vi "CameraSubVI.vi"(2 "Plik wyjsciowy 2":path=path "f:/test.jpg") -> ()   [LabVIEW 2023]
uses:
  <vilib>/userDefined/High Color/IMAQdx.ctl
  <vilib>/vision/driver/NI_Vision_Acquisition_Software.lvlib
panel:
  out "Image 3":T1(plugin-control) caption="Image"
  in  "Zapisz 2":bool
  in  "stop 2":bool
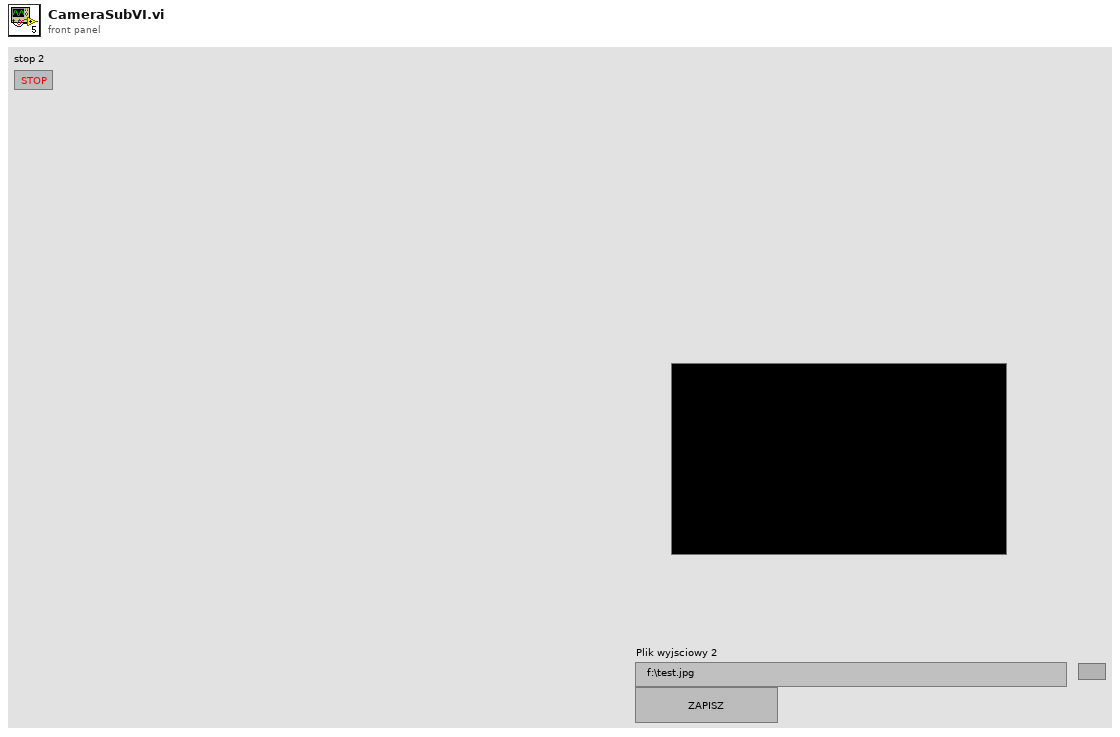
[diagram p1: front panel]
types:
  T1 = typedef "IMAQ Image.ctl" = refnum<image>
  T2 = typedef "IMAQdx.ctl" = refnum<k21>
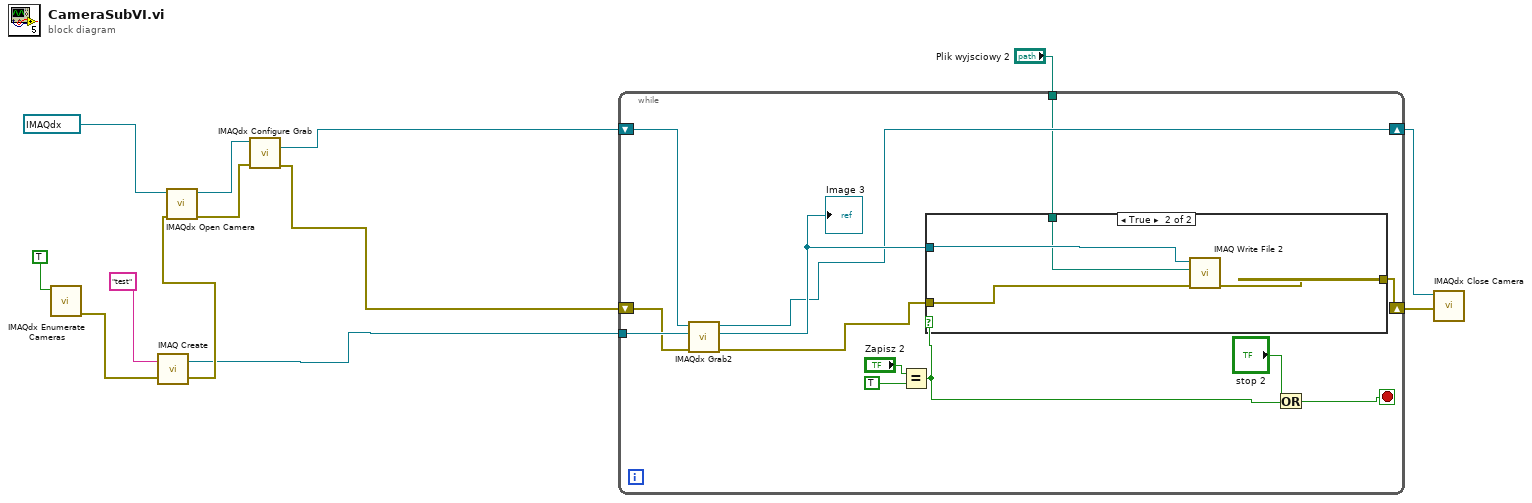
[diagram p0: block diagram]
diagram:
  n1 = call <vilib>:"IMAQdx Enumerate Cameras.vi"("Connected Only? (Yes)"=TRUE) -> ("error out"=w12:errorcluster)  [unwired: 9 in, 1 out]
  n2 = call "IMAQ Create"("Image Name"="test", "error in (no error)"=w12) -> ("New Image"=w8:T1, "error out"=w10:errorcluster)  [unwired: 2 in, 1 out]
  n3 = call <vilib>:"IMAQdx Open Camera.vi"("error in"=w10, "Session In"=T2 "cam0") -> ("error out"=w5:errorcluster, "Session Out"=w6:T2)  [unwired: 1 in, 7 out]
  n4 = call <vilib>:"IMAQdx Configure Grab.vi"("error in"=w5, "Session In"=w6) -> ("error out"=w4:errorcluster, "Session Out"=w3:T2)  [unwired: 8 in]
  n5 = while {
    tunnel: w8 -> [w22]
    shift-right: [w26] -> w9
    shift-left: w4 -> [w19]
    shift-right: [w20] -> w7
    shift-left: w3 -> [w18]
    tunnel: "Plik wyjsciowy 2" -> [w14]
    stop <- w15 stop-if-true
    n6 = call <vilib>:"IMAQdx Grab2.vi"("error in"=w19, "Image In"=w22, "Session In"=w18) -> ("error out"=w23:errorcluster, "Image Out"=w21:T1, "Session Out"=w20:T2)  [unwired: 5 in, 1 out]
    "Image 3" <- w21
    n7 = Equal?(x="Zapisz 2", y=TRUE) -> (x = y?=w17:bool)
    n8 = case shown="True" w17 {
      tunnel: w23 -> [w27 w31]
      tunnel: [w27 w30] -> w26
      tunnel: w21 -> [_ w29]
      tunnel: w14 -> [_ w28]
      frame False {
      }
      frame True {
        n9 = call-poly "IMAQ Write File 2"("error in (no error)"=w31, "File Path"=w28, "Image"=w29) -> ("error out"=w30:errorcluster)  [unwired: 2 in, 6 out]
      }
    }
    n10 = Or(x="stop 2", y=w17) -> (x .or. y?=w15:bool)
  }
  n11 = call <vilib>:"IMAQdx Close Camera.vi"("error in"=w9, "Session In"=w7) -> ()  [unwired: 9 in, 1 out]
